vi "blue plane to processed.vi"(8 "error in (no error)":errorcluster, 11 "Image Src":T1=refnum) -> (0 "error out":errorcluster, 2 "Number of Particles":i32=1, 3 "Image Dst Out":T1, 7 "Number of Particles1":i32=17)   [LabVIEW 2009]
uses:
  <vilib>/vision/Image Controls.llb/IMAQ Image.ctl
  <vilib>/vision/NI_Vision_Development_Module.lvlib
  <vilib>/Analysis/NI_AALBase.lvlib
panel:
  in  "upper limit":dbl(slide)=255.0 min=0.0 max=255.0 step=1.0 scale=0.0..255.0
  in  "lower limit":dbl(slide)=70.0 min=0.0 max=255.0 step=1.0 scale=0.0..255.0
  out "Image Out":T1(plugin-control)
  out "Elongation array 2":T3(array[cluster])=[{"Measurement Parameter"=53, "Range Lower Value"=0, 3.0011306788895187, "Range"=TRUE, "Measurement Type"=FALSE}] {"Measurement Parameter" items=["Center of Mass X", "Center of Mass Y", "First Pixel X", "First Pixel Y", "Bounding Rect Left", "Bounding Rect Top", "Bounding Rect Right", "Bounding Rect Bottom", "Max Feret Diameter Start X", "Max Feret Diameter Start Y", "Max Feret Diameter End X", "Max Feret Diameter End Y", "Max Horiz. Segment Length Left", "Max Horiz. Segment Length Right", "Max Horiz. Segment Length Row", "-", "Bounding Rect Width", "Bounding Rect Height", "Bounding Rect Diagonal", "Perimeter", "Convex Hull Perimeter", "Holes' Perimeter", "Max Feret Diameter", "Equivalent Ellipse Major Axis", "Equivalent Ellipse Minor Axis", "Equivalent Ellipse Minor Axis (Feret)", "Equivalent Rect Long Side", "Equivalent Rect Short Side", "Equivalent Rect Diagonal", "Equivalent Rect Short Side (Feret)", "Average Horiz. Segment Length", "Average Vert. Segment Length", "Hydraulic Radius", "Waddel Disk Diameter", "-", "Area", "Holes' Area", "Particle & Holes' Area", "Convex Hull Area", "Image Area", "-", "Number of Holes", "Number of Horiz. Segments", "Number of Vert. Segments", "-", "Orientation", "Max Feret Diameter Orientation", "-", "% Area/Image Area", "% Area/(Particle & Holes' Area)", "Ratio of Equivalent Ellipse Axes", "Ratio of Equivalent Rect Sides", "-", "Elongation Factor", "Compactness Factor", "Heywood Circularity Factor", "Type Factor", "-", "Sum X", "Sum Y", "Sum XX", "Sum XY", "Sum YY", "Sum XXX", "Sum XXY", "Sum XYY", "Sum YYY", "-", "Moment of Inertia XX", "Moment of Inertia XY", "Moment of Inertia YY", "Moment of Inertia XXX", "Moment of Inertia XXY", "Moment of Inertia XYY", "Moment of Inertia YYY", "Norm. Moment of Inertia XX", "Norm. Moment of Inertia XY", "Norm. Moment of Inertia YY", "Norm. Moment of Inertia XXX", "Norm. Moment of Inertia XXY", "Norm. Moment of Inertia XYY", "Norm. Moment of Inertia YYY", "Hu Moment 1", "Hu Moment 2", "Hu Moment 3", "Hu Moment 4", "Hu Moment 5", "Hu Moment 6", "Hu Moment 7"]}
  out "Elongation Threshold":dbl=3.0011306788895187
  in  "Elongation Multiplier":sgl=1.15
  out "Elongation STV":dbl=0.5914076871600648 format="%0.2f"
  out "Elongation Array":dbl[](array[numeric])=[2.165413533834586, 2.321428571428571, 2.25609756097561, 4.247298919567827, 2.0, 1.6654616659135413, 2.0634920634920633, 2.0178571428571432, 2.0178571428571432, 2.4666666666666663, 3.0526315789473686, 2.0000000000000004, 2.013888888888889, 2.0543032786885242, 2.3566433566433567, 2.031746031746032, 2.7264150943396226]
  out "Elongation Mean":dbl=2.3210118527557024 format="%0.2f"
  out "Particle Measurements (Pixels) 2":dbl[][](array[numeric])=[[2.165413533834586], [2.321428571428571], [2.25609756097561], [4.247298919567827], [2.0], [1.6654616659135413], [2.0634920634920633], [2.0178571428571432], [2.0178571428571432], [2.4666666666666663], [3.0526315789473686], [2.0000000000000004], [2.013888888888889], [2.0543032786885242], [2.3566433566433567], [2.031746031746032], [2.7264150943396226]] format="%.2f"
  out "Particle Measurements (Pixels)":dbl[][](array[numeric])=[[2.165413533834586], [2.321428571428571], [2.25609756097561], [4.247298919567827], [2.0], [1.6654616659135413], [2.0634920634920633], [2.0178571428571432], [2.0178571428571432], [2.4666666666666663], [3.0526315789473686], [2.0000000000000004], [2.013888888888889], [2.0543032786885242], [2.3566433566433567], [2.031746031746032], [2.7264150943396226]] format="%.2f"
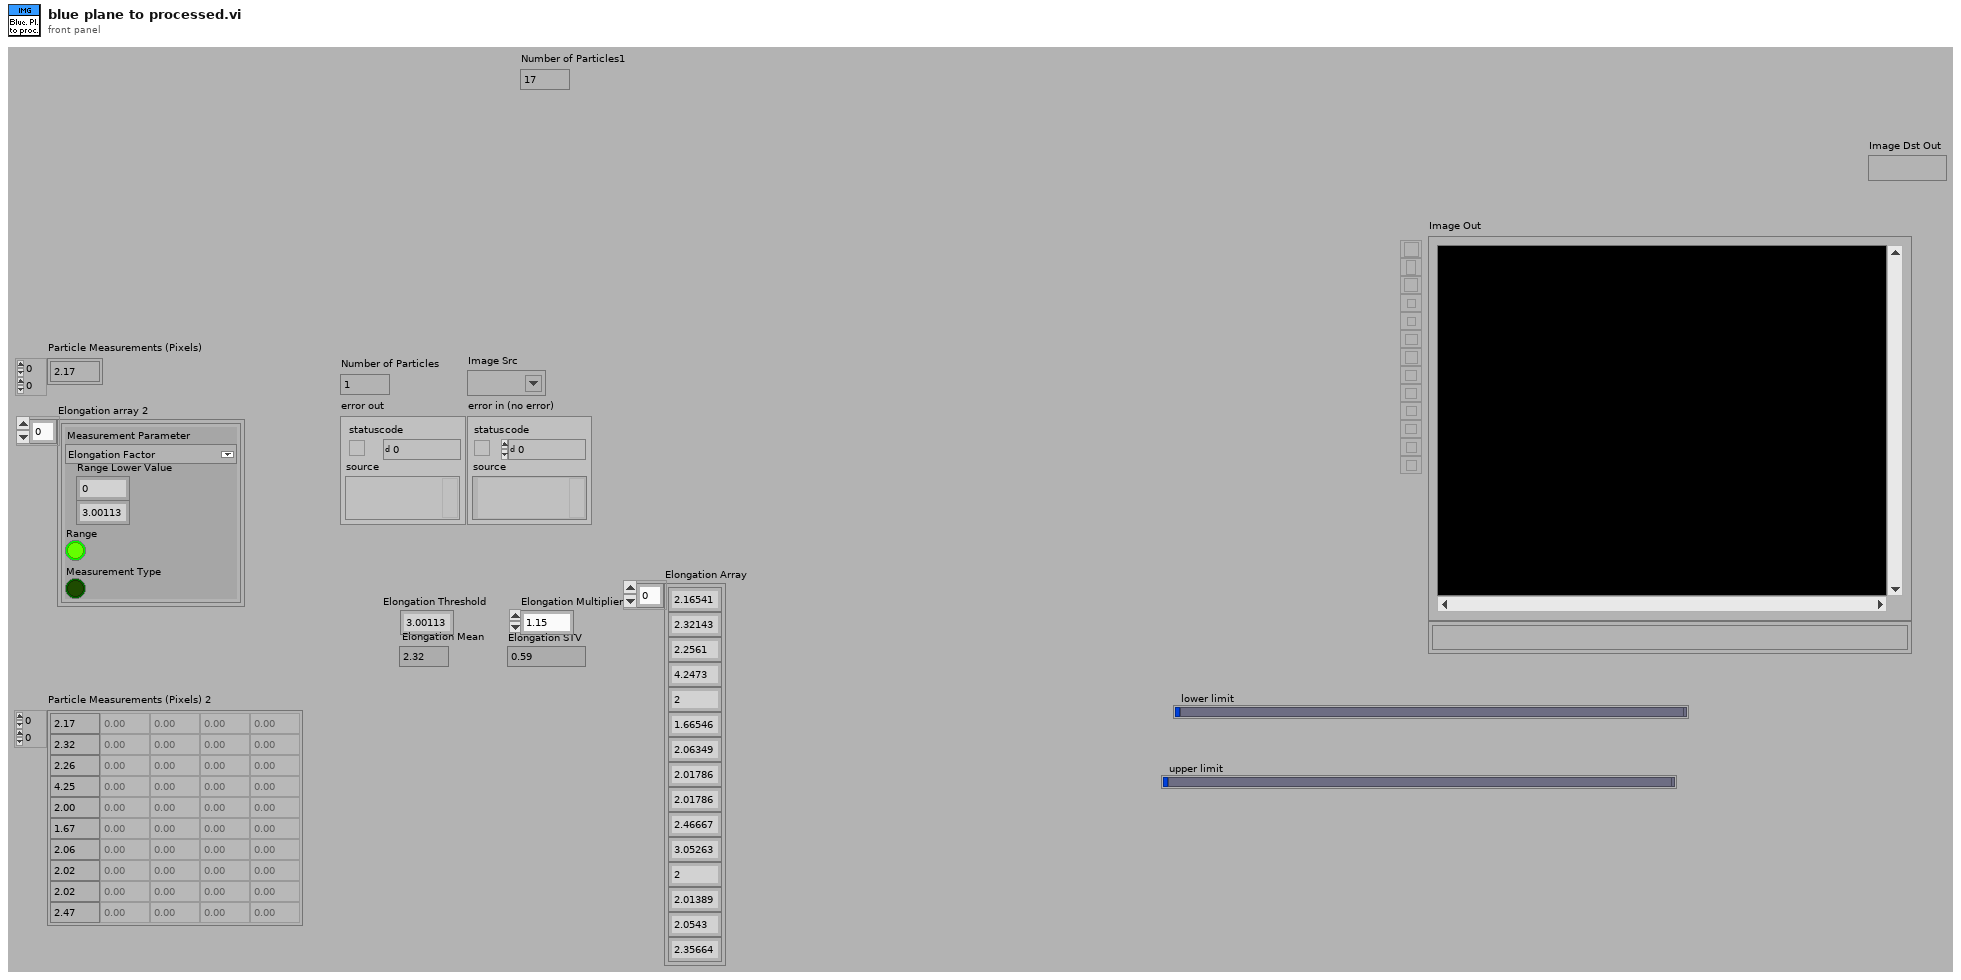
[diagram p1: front panel]
types:
  T1 = typedef "IMAQ Image.ctl" = refnum<image>
  T2 = typedef "Particle Parameters" = i32
  T3 = cluster{"Measurement Parameter":T2, "Range Lower Value":i32, dbl, "Range":bool, "Measurement Type":bool}[]
  T4 = enum32{"AutoM", "Close", "Dilate", "Erode", "Gradient", "Gradient out", "Gradient in", "Hit miss", "Open", "PClose", "POpen", "Thick", "Thin"}
  T5 = typedef "Image Type" = u32
  T6 = cluster{"Measurement Parameter":T2, "Range Lower Value":dbl, "Range Upper Value":dbl, "Range":bool, "Measurement Type":bool}[]
  T7 = enum32{"Linear", "Log", "Exp", "Square", "Square root", "Power X", "Power 1/X"}
  T8 = cluster{"Measurement Parameter":T2, "Range Lower Value":i32, dbl, "Range":bool, "Measurement Type":bool}
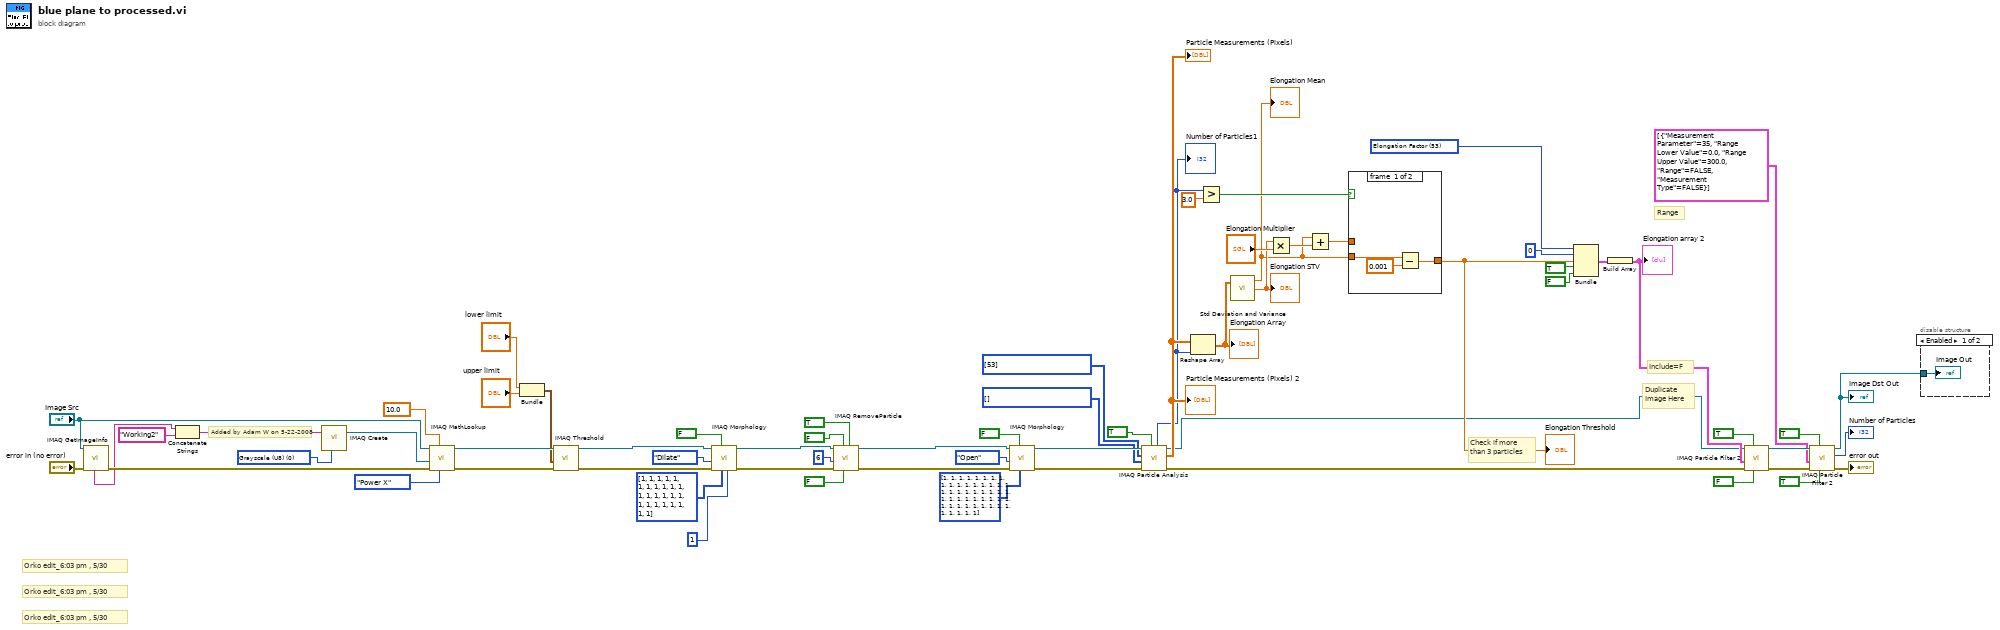
[diagram p0: block diagram]
diagram:
  w19 = T5 0 items=["Grayscale (U8)", "Grayscale (I16)", "Grayscale (SGL)", "Complex (CSG)", "RGB (U32)", "HSL (U32)", "RGB (U64)", "Grayscale (U16)"] ("Image Type")
  w37 = T2 53 items=["Center of Mass X", "Center of Mass Y", "First Pixel X", "First Pixel Y", "Bounding Rect Left", "Bounding Rect Top", "Bounding Rect Right", "Bounding Rect Bottom", "Max Feret Diameter Start X", "Max Feret Diameter Start Y", "Max Feret Diameter End X", "Max Feret Diameter End Y", "Max Horiz. Segment Length Left", "Max Horiz. Segment Length Right", "Max Horiz. Segment Length Row", "-", "Bounding Rect Width", "Bounding Rect Height", "Bounding Rect Diagonal", "Perimeter", "Convex Hull Perimeter", "Holes' Perimeter", "Max Feret Diameter", "Equivalent Ellipse Major Axis", "Equivalent Ellipse Minor Axis", "Equivalent Ellipse Minor Axis (Feret)", "Equivalent Rect Long Side", "Equivalent Rect Short Side", "Equivalent Rect Diagonal", "Equivalent Rect Short Side (Feret)", "Average Horiz. Segment Length", "Average Vert. Segment Length", "Hydraulic Radius", "Waddel Disk Diameter", "-", "Area", "Holes' Area", "Particle & Holes' Area", "Convex Hull Area", "Image Area", "-", "Number of Holes", "Number of Horiz. Segments", "Number of Vert. Segments", "-", "Orientation", "Max Feret Diameter Orientation", "-", "% Area/Image Area", "% Area/(Particle & Holes' Area)", "Ratio of Equivalent Ellipse Axes", "Ratio of Equivalent Rect Sides", "-", "Elongation Factor", "Compactness Factor", "Heywood Circularity Factor", "Type Factor", "-", "Sum X", "Sum Y", "Sum XX", "Sum XY", "Sum YY", "Sum XXX", "Sum XXY", "Sum XYY", "Sum YYY", "-", "Moment of Inertia XX", "Moment of Inertia XY", "Moment of Inertia YY", "Moment of Inertia XXX", "Moment of Inertia XXY", "Moment of Inertia XYY", "Moment of Inertia YYY", "Norm. Moment of Inertia XX", "Norm. Moment of Inertia XY", "Norm. Moment of Inertia YY", "Norm. Moment of Inertia XXX", "Norm. Moment of Inertia XXY", "Norm. Moment of Inertia XYY", "Norm. Moment of Inertia YYY", "Hu Moment 1", "Hu Moment 2", "Hu Moment 3", "Hu Moment 4", "Hu Moment 5", "Hu Moment 6", "Hu Moment 7"] ("Measurement Parameter")
  w45 = T2[] [] items=["Center of Mass X", "Center of Mass Y", "First Pixel X", "First Pixel Y", "Bounding Rect Left", "Bounding Rect Top", "Bounding Rect Right", "Bounding Rect Bottom", "Max Feret Diameter Start X", "Max Feret Diameter Start Y", "Max Feret Diameter End X", "Max Feret Diameter End Y", "Max Horiz. Segment Length Left", "Max Horiz. Segment Length Right", "Max Horiz. Segment Length Row", "-", "Bounding Rect Width", "Bounding Rect Height", "Bounding Rect Diagonal", "Perimeter", "Convex Hull Perimeter", "Holes' Perimeter", "Max Feret Diameter", "Equivalent Ellipse Major Axis", "Equivalent Ellipse Minor Axis", "Equivalent Ellipse Minor Axis (Feret)", "Equivalent Rect Long Side", "Equivalent Rect Short Side", "Equivalent Rect Diagonal", "Equivalent Rect Short Side (Feret)", "Average Horiz. Segment Length", "Average Vert. Segment Length", "Hydraulic Radius", "Waddel Disk Diameter", "-", "Area", "Holes' Area", "Particle & Holes' Area", "Convex Hull Area", "Image Area", "-", "Number of Holes", "Number of Horiz. Segments", "Number of Vert. Segments", "-", "Orientation", "Max Feret Diameter Orientation", "-", "% Area/Image Area", "% Area/(Particle & Holes' Area)", "Ratio of Equivalent Ellipse Axes", "Ratio of Equivalent Rect Sides", "-", "Elongation Factor", "Compactness Factor", "Heywood Circularity Factor", "Type Factor", "-", "Sum X", "Sum Y", "Sum XX", "Sum XY", "Sum YY", "Sum XXX", "Sum XXY", "Sum XYY", "Sum YYY", "-", "Moment of Inertia XX", "Moment of Inertia XY", "Moment of Inertia YY", "Moment of Inertia XXX", "Moment of Inertia XXY", "Moment of Inertia XYY", "Moment of Inertia YYY", "Norm. Moment of Inertia XX", "Norm. Moment of Inertia XY", "Norm. Moment of Inertia YY", "Norm. Moment of Inertia XXX", "Norm. Moment of Inertia XXY", "Norm. Moment of Inertia XYY", "Norm. Moment of Inertia YYY", "Hu Moment 1", "Hu Moment 2", "Hu Moment 3", "Hu Moment 4", "Hu Moment 5", "Hu Moment 6", "Hu Moment 7"] ("Real-World Measurements")
  w46 = T2[] [53] items=["Center of Mass X", "Center of Mass Y", "First Pixel X", "First Pixel Y", "Bounding Rect Left", "Bounding Rect Top", "Bounding Rect Right", "Bounding Rect Bottom", "Max Feret Diameter Start X", "Max Feret Diameter Start Y", "Max Feret Diameter End X", "Max Feret Diameter End Y", "Max Horiz. Segment Length Left", "Max Horiz. Segment Length Right", "Max Horiz. Segment Length Row", "-", "Bounding Rect Width", "Bounding Rect Height", "Bounding Rect Diagonal", "Perimeter", "Convex Hull Perimeter", "Holes' Perimeter", "Max Feret Diameter", "Equivalent Ellipse Major Axis", "Equivalent Ellipse Minor Axis", "Equivalent Ellipse Minor Axis (Feret)", "Equivalent Rect Long Side", "Equivalent Rect Short Side", "Equivalent Rect Diagonal", "Equivalent Rect Short Side (Feret)", "Average Horiz. Segment Length", "Average Vert. Segment Length", "Hydraulic Radius", "Waddel Disk Diameter", "-", "Area", "Holes' Area", "Particle & Holes' Area", "Convex Hull Area", "Image Area", "-", "Number of Holes", "Number of Horiz. Segments", "Number of Vert. Segments", "-", "Orientation", "Max Feret Diameter Orientation", "-", "% Area/Image Area", "% Area/(Particle & Holes' Area)", "Ratio of Equivalent Ellipse Axes", "Ratio of Equivalent Rect Sides", "-", "Elongation Factor", "Compactness Factor", "Heywood Circularity Factor", "Type Factor", "-", "Sum X", "Sum Y", "Sum XX", "Sum XY", "Sum YY", "Sum XXX", "Sum XXY", "Sum XYY", "Sum YYY", "-", "Moment of Inertia XX", "Moment of Inertia XY", "Moment of Inertia YY", "Moment of Inertia XXX", "Moment of Inertia XXY", "Moment of Inertia XYY", "Moment of Inertia YYY", "Norm. Moment of Inertia XX", "Norm. Moment of Inertia XY", "Norm. Moment of Inertia YY", "Norm. Moment of Inertia XXX", "Norm. Moment of Inertia XXY", "Norm. Moment of Inertia XYY", "Norm. Moment of Inertia YYY", "Hu Moment 1", "Hu Moment 2", "Hu Moment 3", "Hu Moment 4", "Hu Moment 5", "Hu Moment 6", "Hu Moment 7"] ("Pixel Measurements")
  # "Orko edit_6:03 pm , 5/30"
  # "Orko edit_6:03 pm , 5/30"
  # "Orko edit_6:03 pm , 5/30"
  # "Range"
  # "Include=F"
  # "Added by Adam W on 5-22-2008"
  # "Check if more\nthan 3 particles"
  # "Duplicate\nImage Here"
  n1 = call "IMAQ GetImageInfo"("error in (no error)"="error in (no error)", "Image"="Image Src") -> ("error out"=w53:errorcluster, "Image Name"=w51:string)  [unwired: 8 out]
  n2 = Concatenate Strings(w51, "Working2" ("Image Name")) -> (w52:string)
  n3 = call "IMAQ Create"("Image Name"=w52, "Image Type"=w19) -> ("New Image"=w20:T1)  [unwired: 2 in, 2 out]
  n4 = call "IMAQ MathLookup"("Operator"=T7."Power X", "X Value"=sgl 10.0, "error in (no error)"=w53, "Image Dst"=w20, "Image Src"="Image Src") -> ("error out"=w64:errorcluster, "Image Dst Out"=w2:T1)  [unwired: 2 in, 3 out]
  n5 = Bundle("lower limit"="lower limit", "upper limit"="upper limit") -> (w1:cluster{"lower limit":dbl, "upper limit":dbl})  [unwired: 1 out]
  n6 = call "IMAQ Threshold"("error in (no error)"=w64, "Range"=w1, "Image Src"=w2) -> ("error out"=w61:errorcluster, "Image Dst Out"=w49:T1)  [unwired: 3 in, 4 out]
  n7 = call "IMAQ Morphology"("Number of iterations (1)"=1, "Structuring Element"=i32[][] [[1, 1, 1, 1, 1], [1, 1, 1, 1, 1], [1, 1, 1, 1, 1], [1, 1, 1, 1, 1], [1, 1, 1, 1, 1]], "Square/Hexa (Square)"=FALSE, "error in (no error)"=w61, "Operation"=T4."Dilate", "Image Src"=w49) -> ("error out"=w60:errorcluster, "Image Dst Out"=w57:T1)  [unwired: 1 in, 3 out]
  n8 = call "IMAQ RemoveParticle"("Connectivity 4/8 (8)"=TRUE, "Low Pass/High Pass (Low)"=FALSE, "Square/Hexa (Square)"=FALSE, "error in (no error)"=w60, "Number of Erosion"=6, "Image Src"=w57) -> ("error out"=w59:errorcluster, "Image Dst Out"=w58:T1)  [unwired: 4 in]
  n9 = call "IMAQ Morphology"("Structuring Element"=i32[][] [[1, 1, 1, 1, 1, 1, 1], [1, 1, 1, 1, 1, 1, 1], [1, 1, 1, 1, 1, 1, 1], [1, 1, 1, 1, 1, 1, 1], [1, 1, 1, 1, 1, 1, 1], [1, 1, 1, 1, 1, 1, 1], [1, 1, 1, 1, 1, 1, 1]], "Square/Hexa (Square)"=FALSE, "error in (no error)"=w59, "Operation"=T4."Open", "Image Src"=w58) -> ("error out"=w55:errorcluster, "Image Dst Out"=w56:T1)  [unwired: 2 in, 3 out]
  n10 = call "IMAQ Particle Analysis"("Connectivity 4/8 (8)"=TRUE, "error in (no error)"=w55, "Real-World Measurements"=w45, "Pixel Measurements"=w46, "Image"=w56) -> ("error out"=w21:errorcluster, "Particle Measurements (Pixels)"=w43:dbl[][], "Image Out (duplicate)"=w18:T1, "Number of Particles"=w31:i32)  [unwired: 3 out]
  "Particle Measurements (Pixels)" <- w43
  "Particle Measurements (Pixels) 2" <- w43
  "Number of Particles1" <- w31
  n11 = Reshape Array(w43, w31) -> (w42:dbl[])
  "Elongation Array" <- w42
  n12 = Greater?(x=w31, y=3.0) -> (0:w30:bool)
  n13 = call <vilib>:"Std Deviation and Variance.vi"("X"=w42) -> ("mean"=w28:dbl, "standard deviation"=w39:dbl)  [unwired: 1 in, 1 out]
  "Elongation Mean" <- w28
  "Elongation STV" <- w39
  n14 = Multiply(x=w39, y="Elongation Multiplier") -> (x*y=w41:dbl)
  n15 = Add(x=w28, y=w41) -> (x+y=w29:dbl)
  n16 = case shown="False" w30 {
    tunnel: w29 -> [_ w70]
    tunnel: [w67 w70] -> w27
    tunnel: w28 -> [w69 _]
    frame #0 {
      n17 = Subtract(x=w69, y=0.001) -> (x-y=w67:dbl)
    }
    frame #1 {
    }
  }
  "Elongation Threshold" <- w27
  n18 = Bundle("Measurement Parameter"=w37, "Range Lower Value"=0, w27, "Range"=TRUE, "Measurement Type"=FALSE) -> (w34:T8)  [unwired: 1 out]
  n19 = Build Array(w34) -> (w33:T3)
  "Elongation array 2" <- w33
  n20 = call "IMAQ Particle Filter 2"("Keep/Remove Particles (F)"=FALSE ("Keep/Remove Particles"), "Connectivity 4/8 (8)"=TRUE, "error in (no error)"=w21, "Selection Values"=w33, "Image Src"=w18) -> ("error out"=w25:errorcluster, "Image Dst Out"=w26:T1)  [unwired: 3 in, 2 out]
  n21 = call "IMAQ Particle Filter 2"("Keep/Remove Particles (F)"=TRUE ("Keep/Remove Particles"), "Connectivity 4/8 (8)"=TRUE, "error in (no error)"=w25, "Selection Values"=T6 [{"Measurement Parameter"=35, "Range Lower Value"=0.0, "Range Upper Value"=300.0, "Range"=FALSE, "Measurement Type"=FALSE}], "Image Src"=w26) -> ("error out"=→"error out":errorcluster, "Number of Particles"=→"Number of Particles":i32, "Image Dst Out"=w17:T1)  [unwired: 3 in, 1 out]
  "Image Dst Out" <- w17
  n22 = disable-structure shown="Enabled" {
    disable-tunnel: w17 -> [w71 _]
    frame #0 {
      "Image Out" <- w71
    }
    frame #1 {
    }
  }
